vi "Clean XY Graph.vi"(11 "XY Graph Reference In":refnum<vi>) -> (3 "XY Graph Reference Out":refnum<vi>)   [LabVIEW 2022 SP3]
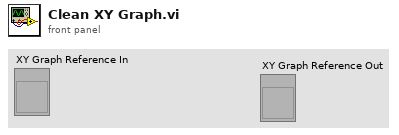
[diagram p1: front panel]
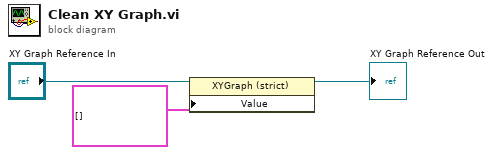
[diagram p0: block diagram]
diagram:
  n1 = property class="XYGraph (strict)"(reference="XY Graph Reference In", "Value"=cluster{"Wavenumber":dbl[], "Data":dbl[]}[] []) -> (reference out=→"XY Graph Reference Out":refnum<vi>)  [unwired: 1 in, 1 out]
